vi "CCE MGLD PMJD PF SubVI04.vi"(8 "tapa?":bool, 9 "y":sgl=0.75, 10 "x":sgl=0.75, 11 "Image 2":T1) -> (2 "Array":bool[](array[boolean]), 3 "Image":T1(plugin-control))   [LabVIEW 2020]
doc: "Ceballos Conde Emanuel Meneses Gutiérrez Luis David Pineda Méndez Job Daniel 4MV6 Sistemas de visión artificial 2022/1 \nEste vi obtiene el nivel de liquido oscuro presente en una botella , permite obtener hasta 4 resultados distintos los cuales son: vacío, bajo , medio y alto representados por un arreglo de elementos boleanos"
uses:
  <vilib>/vision/Image Controls.llb/IMAQ Image.ctl
  <vilib>/vision/NI_Vision_Development_Module.lvlib
panel:
  out "Color Spectrum":dbl[](array[numeric]) format="%.2f"
  # "Ceballos Conde Emanuel   -  Meneses Gutiérrez Luis David   -  Pineda Méndez Job Daniel 4MV6 Sistemas de visión artificial  2022/1             SubVI04"
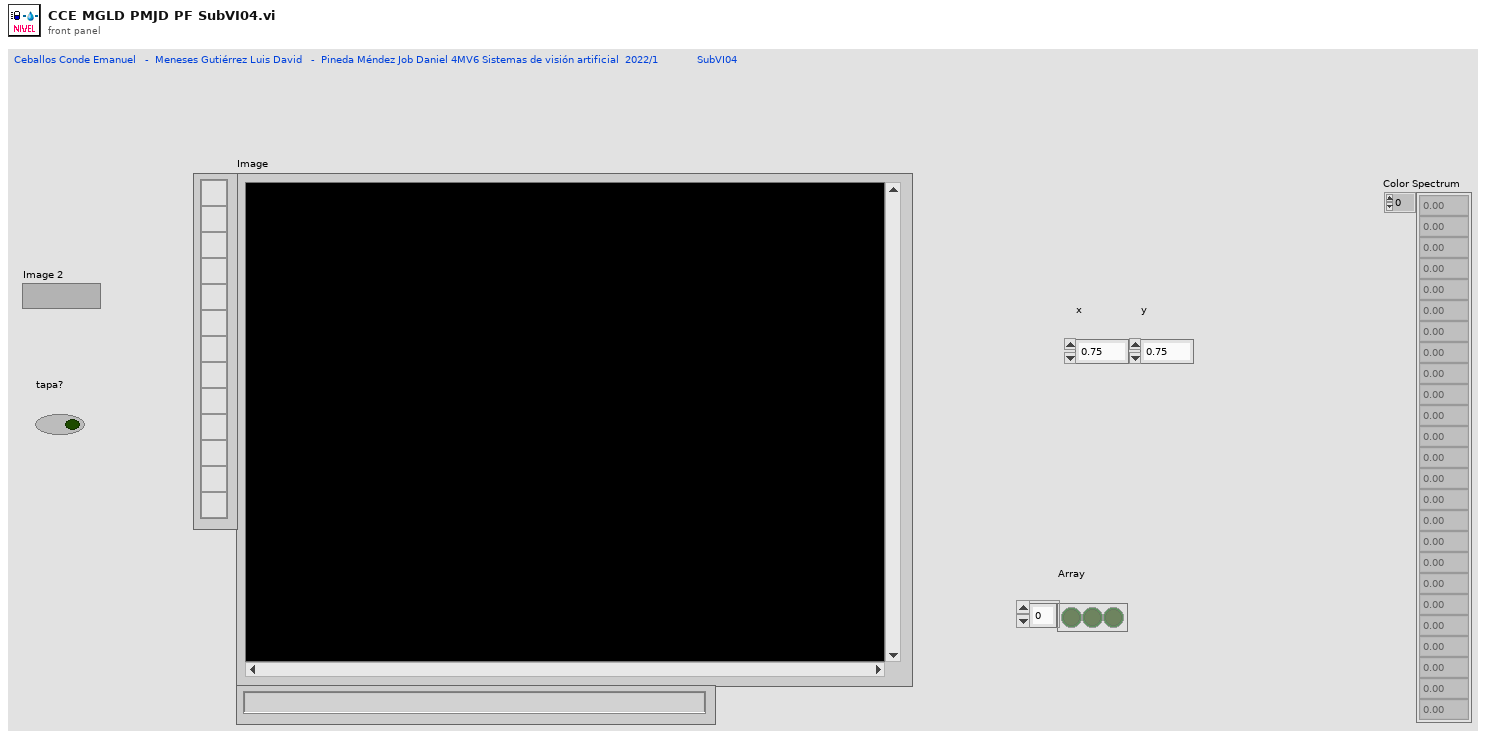
[diagram p1: front panel]
types:
  T1 = typedef "IMAQ Image.ctl" = refnum<image>
  T2 = typedef "ROI Descriptor" = cluster{"Global Rectangle":i32[], "Contours":cluster{"ID":enum32{"External", "Internal"}, "Type":u32, "Coordinates":i32[]}[]}
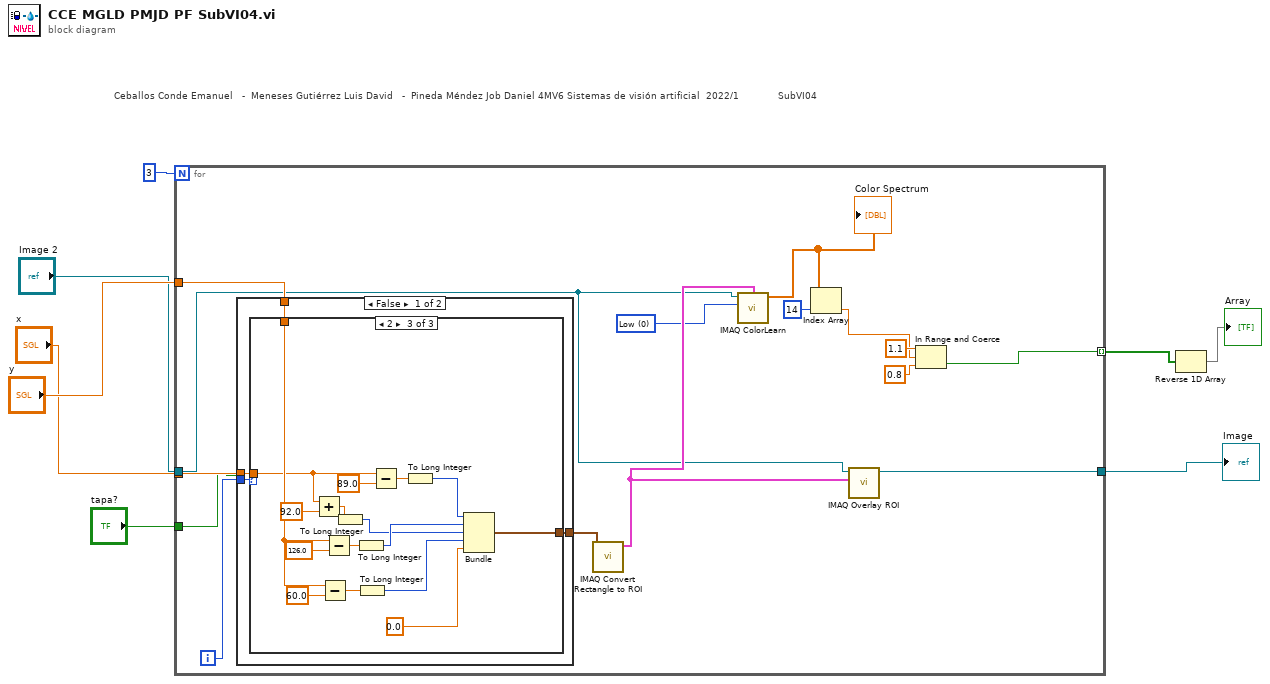
[diagram p0: block diagram]
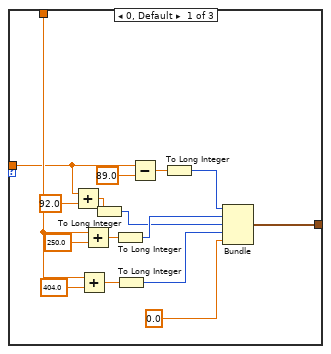
[diagram p2: hidden frame]
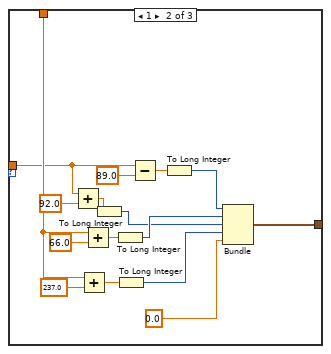
[diagram p3: hidden frame]
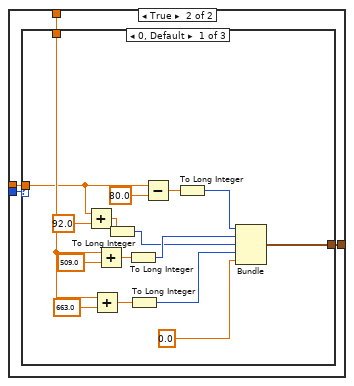
[diagram p4: hidden frame]
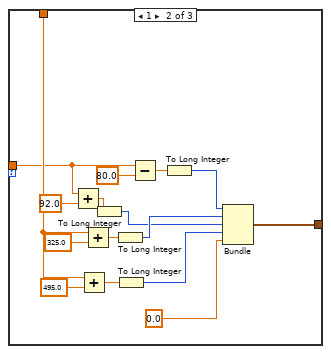
[diagram p5: hidden frame]
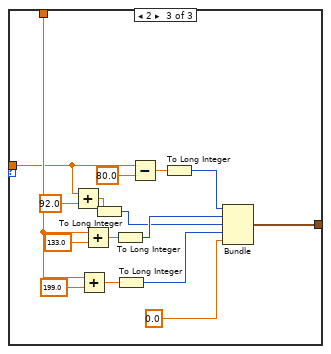
[diagram p6: hidden frame]
diagram:
  # "Ceballos Conde Emanuel   -  Meneses Gutiérrez Luis David   -  Pineda Méndez Job Daniel 4MV6 Sistemas de visión artificial  2022/1             SubVI04"
  n1 = for {
    N: 3 -> [_]
    tunnel: [w19] -> w3 mode=indexing
    tunnel: "y" -> [w17]
    tunnel: "x" -> [w16]
    tunnel: "tapa?" -> [w9]
    tunnel: "Image 2" -> [w12]
    tunnel: [w14] -> w6
    i -> [w10]
    w11 = u32 0 items=["Low", "Medium", "High"] ("Color Sensitivity")
    n2 = case shown="False" w9 {
      tunnel: w17 -> [w27 w79]
      tunnel: w16 -> [w26 w78]
      tunnel: [w25 w77] -> w15
      tunnel: w10 -> [w24 w76]
      frame False {
        n3 = case shown="2" w24 {
          tunnel: w27 -> [w43 w59 w75]
          tunnel: w26 -> [w42 w58 w74]
          tunnel: [w35 w51 w67] -> w25
          frame 0, Default {
            n4 = Add(x=w42, y=sgl 92.0) -> (x+y=w38:sgl)
            n5 = Add(x=w43, y=sgl 404.0) -> (x+y=w39:sgl)
            n6 = Add(x=w43, y=sgl 250.0) -> (x+y=w40:sgl)
            n7 = To Long Integer(number=w38) -> (32bit integer=w29:i32)
            n8 = To Long Integer(number=w40) -> (32bit integer=w30:i32)
            n9 = To Long Integer(number=w39) -> (32bit integer=w28:i32)
            n10 = Subtract(x=w42, y=sgl 89.0) -> (x-y=w41:sgl)
            n11 = To Long Integer(number=w41) -> (32bit integer=w36:i32)
            n12 = Bundle(w36, w30, w29, w28, 0.0) -> (w35:cluster{i32, i32, i32, i32, dbl})  [unwired: 1 in]
          }
          frame 1 {
            n13 = Add(x=w58, y=sgl 92.0) -> (x+y=w54:sgl)
            n14 = Add(x=w59, y=sgl 237.0) -> (x+y=w55:sgl)
            n15 = Add(x=w59, y=sgl 66.0) -> (x+y=w56:sgl)
            n16 = To Long Integer(number=w54) -> (32bit integer=w45:i32)
            n17 = To Long Integer(number=w56) -> (32bit integer=w46:i32)
            n18 = To Long Integer(number=w55) -> (32bit integer=w44:i32)
            n19 = Subtract(x=w58, y=sgl 89.0) -> (x-y=w57:sgl)
            n20 = To Long Integer(number=w57) -> (32bit integer=w52:i32)
            n21 = Bundle(w52, w46, w45, w44, 0.0) -> (w51:cluster{i32, i32, i32, i32, dbl})  [unwired: 1 in]
          }
          frame 2 {
            n22 = Add(x=w74, y=sgl 92.0) -> (x+y=w70:sgl)
            n23 = Subtract(x=w75, y=sgl 60.0) -> (x-y=w71:sgl)
            n24 = Subtract(x=w75, y=sgl 126.0) -> (x-y=w72:sgl)
            n25 = To Long Integer(number=w70) -> (32bit integer=w61:i32)
            n26 = To Long Integer(number=w72) -> (32bit integer=w62:i32)
            n27 = To Long Integer(number=w71) -> (32bit integer=w60:i32)
            n28 = Subtract(x=w74, y=sgl 89.0) -> (x-y=w73:sgl)
            n29 = To Long Integer(number=w73) -> (32bit integer=w68:i32)
            n30 = Bundle(w68, w62, w61, w60, 0.0) -> (w67:cluster{i32, i32, i32, i32, dbl})  [unwired: 1 in]
          }
        }
      }
      frame True {
        n31 = case shown="0, Default" w76 {
          tunnel: w79 -> [w95 w111 w127]
          tunnel: w78 -> [w94 w110 w126]
          tunnel: [w87 w103 w119] -> w77
          frame 0, Default {
            n32 = Add(x=w94, y=sgl 92.0) -> (x+y=w90:sgl)
            n33 = Add(x=w95, y=sgl 663.0) -> (x+y=w91:sgl)
            n34 = Add(x=w95, y=sgl 509.0) -> (x+y=w92:sgl)
            n35 = To Long Integer(number=w90) -> (32bit integer=w81:i32)
            n36 = To Long Integer(number=w92) -> (32bit integer=w82:i32)
            n37 = To Long Integer(number=w91) -> (32bit integer=w80:i32)
            n38 = Subtract(x=w94, y=sgl 80.0) -> (x-y=w93:sgl)
            n39 = To Long Integer(number=w93) -> (32bit integer=w88:i32)
            n40 = Bundle(w88, w82, w81, w80, 0.0) -> (w87:cluster{i32, i32, i32, i32, dbl})  [unwired: 1 in]
          }
          frame 1 {
            n41 = Add(x=w110, y=sgl 92.0) -> (x+y=w106:sgl)
            n42 = Add(x=w111, y=sgl 495.0) -> (x+y=w107:sgl)
            n43 = Add(x=w111, y=sgl 325.0) -> (x+y=w108:sgl)
            n44 = To Long Integer(number=w106) -> (32bit integer=w97:i32)
            n45 = To Long Integer(number=w108) -> (32bit integer=w98:i32)
            n46 = To Long Integer(number=w107) -> (32bit integer=w96:i32)
            n47 = Subtract(x=w110, y=sgl 80.0) -> (x-y=w109:sgl)
            n48 = To Long Integer(number=w109) -> (32bit integer=w104:i32)
            n49 = Bundle(w104, w98, w97, w96, 0.0) -> (w103:cluster{i32, i32, i32, i32, dbl})  [unwired: 1 in]
          }
          frame 2 {
            n50 = Add(x=w126, y=sgl 92.0) -> (x+y=w122:sgl)
            n51 = Add(x=w127, y=sgl 199.0) -> (x+y=w123:sgl)
            n52 = Add(x=w127, y=sgl 133.0) -> (x+y=w124:sgl)
            n53 = To Long Integer(number=w122) -> (32bit integer=w113:i32)
            n54 = To Long Integer(number=w124) -> (32bit integer=w114:i32)
            n55 = To Long Integer(number=w123) -> (32bit integer=w112:i32)
            n56 = Subtract(x=w126, y=sgl 80.0) -> (x-y=w125:sgl)
            n57 = To Long Integer(number=w125) -> (32bit integer=w120:i32)
            n58 = Bundle(w120, w114, w113, w112, 0.0) -> (w119:cluster{i32, i32, i32, i32, dbl})  [unwired: 1 in]
          }
        }
      }
    }
    n59 = call "IMAQ Convert Rectangle to ROI"("Rectangle"=w15) -> ("ROI Descriptor"=w13:T2)  [unwired: 8 in, 1 out]
    n60 = call "IMAQ ColorLearn"("ROI Descriptor"=w13, "Image"=w12, "Color Sensitivity"=w11) -> ("Color Spectrum"=w23:dbl[])  [unwired: 5 in, 1 out]
    "Color Spectrum" <- w23
    n61 = Index Array(array=w23, index=14) -> (element=w18:dbl)
    n62 = call "IMAQ Overlay ROI"("ROI Descriptor"=w13, "Image"=w12) -> ("Image Out"=w14:T1)  [unwired: 8 in, 1 out]
    n63 = In Range and Coerce(upper limit=1.1, x=w18, lower limit=0.8) -> (In Range?=w19:bool)  [unwired: 1 out]
  }
  "Image" <- w6
  n64 = Reverse 1D Array(array=w3) -> (reversed array=→"Array":bool[])
